vi "check_for_reboot_loop.vi"(8 "error in (no error)":errorcluster caption="错误输入（无错误）") -> (0 "error out":errorcluster caption="错误输出", 2 "Start in Safe Mode?":bool caption="在安全模式中启动？")   [LabVIEW 2015]
uses:
  globals/global_configuration_options.vi
  <vilib>/Utility/file.llb/Read Delimited Spreadsheet (string).vi
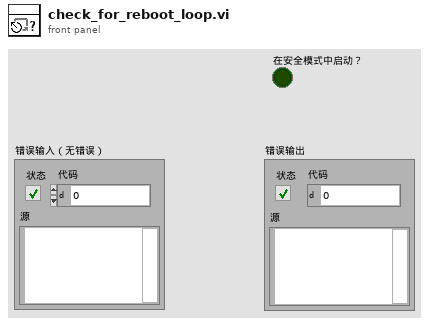
[diagram p1: front panel]
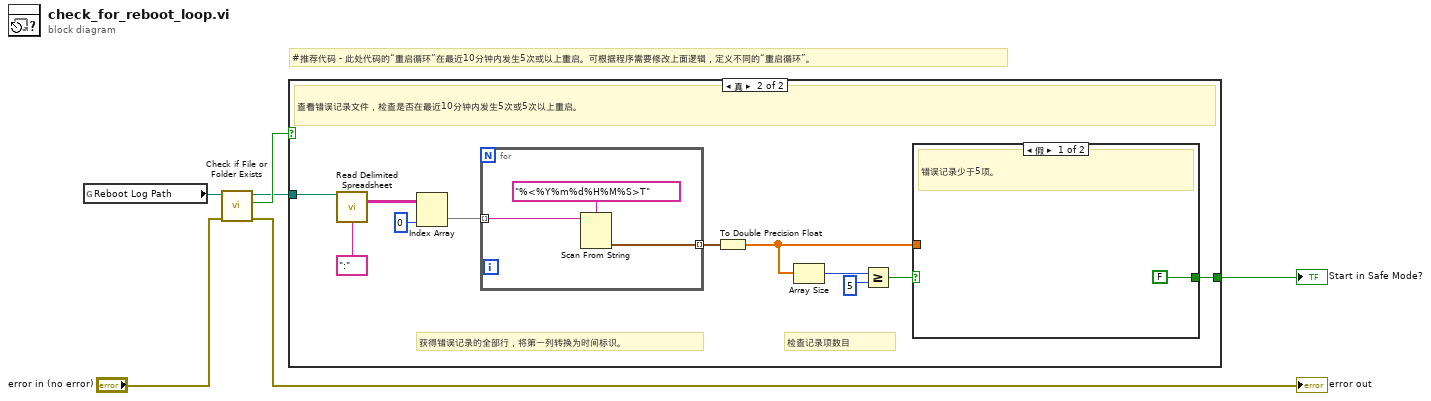
[diagram p0: block diagram]
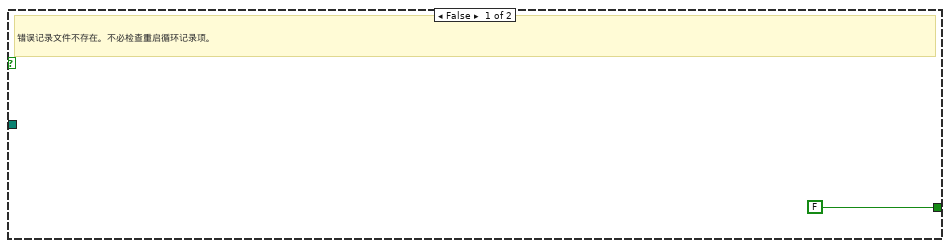
[diagram p2: hidden frame]
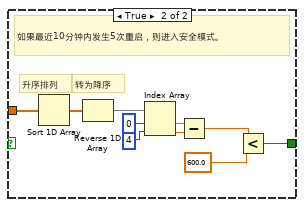
[diagram p3: hidden frame]
diagram:
  # "#推荐代码 - 此处代码的“重启循环”在最近10分钟内发生5次或以上重启。可根据程序需要修改上面逻辑，定义不同的“重启循环”。"
  n1 = global read "global_configuration_options.vi" "Reboot Log Path"() -> (w1:path)
  n2 = call <vilib>:"Check if File or Folder Exists.vi"("error in (no error)"="error in (no error)", "path"=w1) -> ("error out"=→"error out":errorcluster, "file or folder exists?"=w4:bool, "dup path"=w3:path)  [unwired: 7 in]
  n3 = case shown="真" w4 {
    tunnel: w3 -> [_ w11]
    tunnel: [FALSE w16] -> w2
    frame False {
      # "错误记录文件不存在。不必检查重启循环记录项。"
    }
    frame True {
      # "检查记录项数目"
      # "获得错误记录的全部行，将第一列转换为时间标识。"
      # "查看错误记录文件，检查是否在最近10分钟内发生5次或5次以上重启。"
      n4 = call-poly <vilib>:"Read Delimited Spreadsheet.vi"("file path (dialog if empty)"=w11, "delimiter (\\t)"=":") -> ("all rows"=w10:string[][])  [unwired: 8 in, 5 out]
      n5 = Index Array(array=w10, index (col)=0 ("disabled index (col)")) -> (element=w8:string[])  [unwired: 1 in]
      n6 = for {
        tunnel: w8 -> [w32] mode=indexing
        tunnel: [w31] -> w17 mode=indexing
        n7 = Scan From String(format string="%<%Y%m%d%H%M%S>T", input string=w32) -> (output 1=w31:timestamp)  [unwired: 3 in, 3 out]
      }
      n8 = To Double Precision Float(number=w17) -> (double precision float=w15:dbl[])
      n9 = Array Size(array=w15) -> (size(s)=w14:i32)
      n10 = Greater Or Equal?(x=w14, y=5) -> (x >= y?=w12:bool)
      n11 = case shown="假" w12 {
        tunnel: [FALSE w21] -> w16
        tunnel: w15 -> [_ w20]
        frame False {
          # "错误记录少于5项。"
        }
        frame True {
          # "转为降序"
          # "升序排列"
          # "如果最近10分钟内发生5次重启，则进入安全模式。"
          n12 = Sort 1D Array(array=w20) -> (sorted array=w29:dbl[])
          n13 = Reverse 1D Array(array=w29) -> (reversed array=w28:dbl[])
          n14 = Index Array(array=w28, index #1=0 ("index"), index #2=4 ("index")) -> (element #1=w25:dbl, element #2=w24:dbl)
          n15 = Subtract(x=w25, y=w24) -> (x-y=w23:dbl)
          n16 = Less?(x=w23, y=600.0) -> (x < y?=w21:bool)
        }
      }
    }
  }
  "Start in Safe Mode?" <- w2
